vi "serial_disconnect.vi"(7 "serial_disconnect":bool, 8 "error in":errorcluster, 9 "serial_connected in":bool, 11 "VISA Refnum in":refnum<visa-resource-name>) -> (0 "error out":errorcluster, 1 "serial_connected_out":bool)   [LabVIEW 2025]
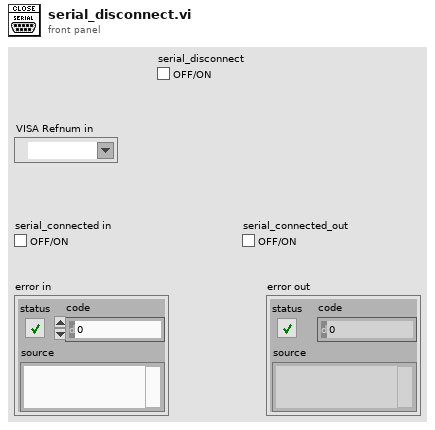
[diagram p1: front panel]
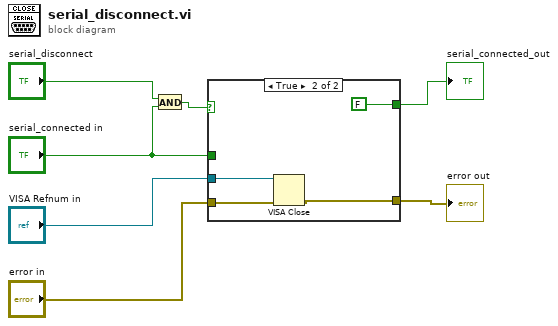
[diagram p0: block diagram]
diagram:
  n1 = And(x="serial_disconnect", y="serial_connected in") -> (x .and. y?=w4:bool)
  n2 = case shown="True" w4 {
    tunnel: "VISA Refnum in" -> [_ w13]
    tunnel: "error in" -> [w8 w12]
    tunnel: [w9 FALSE] -> w5
    tunnel: "serial_connected in" -> [w9 _]
    tunnel: [w8 w10] -> w1
    frame False {
    }
    frame True {
      n3 = VISA Close(VISA resource name=w13, error in (no error)=w12) -> (error out=w10:errorcluster)
    }
  }
  "serial_connected_out" <- w5
  "error out" <- w1
